vi "x-axis.vi"(8 "error in (no error)":errorcluster, 11 "Wavelength iHR320 in":refnum<class "Wavelength iHR320.lvclass">) -> (0 "error out":errorcluster, 1 "Label":string, 2 "Unit":string, 3 "Wavelength iHR320 out":refnum<class "Wavelength iHR320.lvclass">)   [LabVIEW 2012, in "Wavelength iHR320.lvclass"]
uses:
  Wavelength iHR320.lvclass
  Scanner/Scanner.lvclass
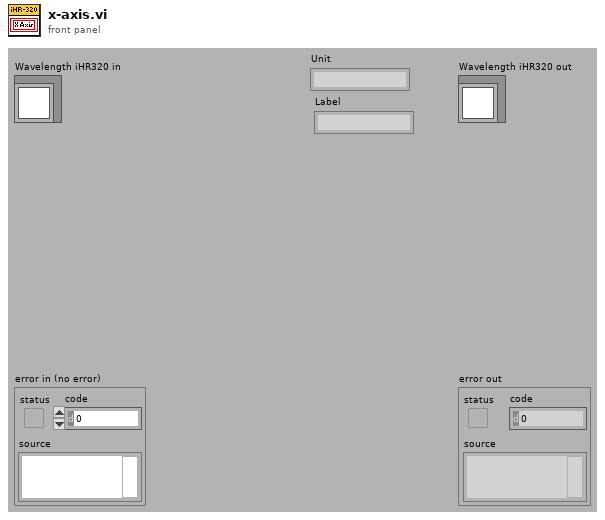
[diagram p1: front panel]
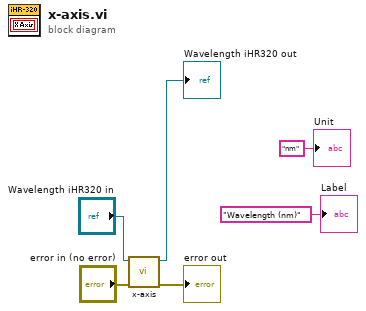
[diagram p0: block diagram]
diagram:
  n1 = call-parent "x-axis.vi"("error in (no error)"="error in (no error)", "Scanner in"="Wavelength iHR320 in") -> ("error out"=→"error out":errorcluster, "Scanner out"=→"Wavelength iHR320 out":refnum<class "Wavelength iHR320.lvclass">)  [unwired: 6 in, 2 out]
  "Label" <- "Wavelength (nm)" ("Label")
  "Unit" <- "nm" ("Unit")
